vi "Read Event Details.vi"(1 "path":path, 2 "OK Button":bool, 3 "Event Name":string) -> (0 "text":string)   [LabVIEW 2014]
panel:
  out "error out":errorcluster
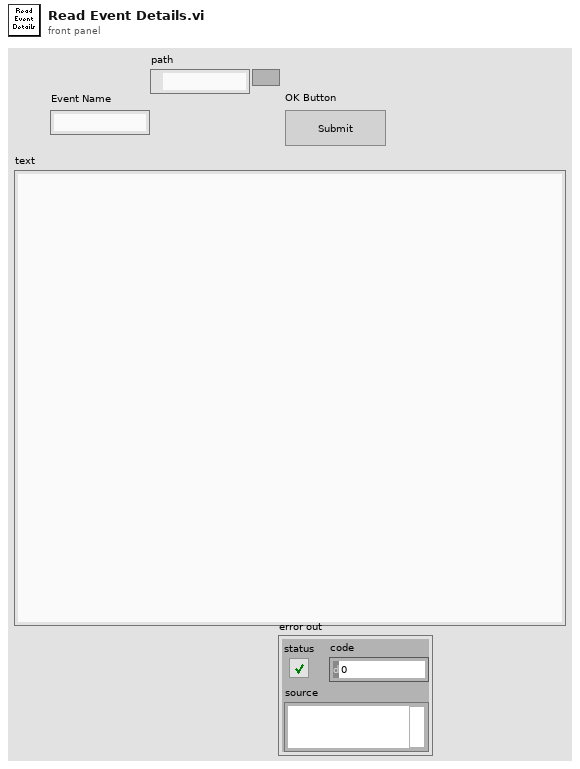
[diagram p1: front panel]
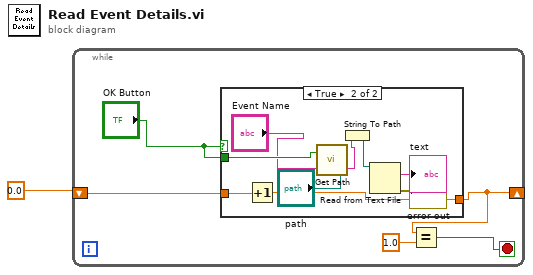
[diagram p0: block diagram]
diagram:
  n1 = while {
    shift-right: [w4] -> _
    shift-left: 0.0 ("Numeric") -> [w6]
    stop <- w5 stop-if-true
    n2 = case shown="True" "OK Button" {
      tunnel: w6 -> [w7 w14]
      tunnel: [w7 w13] -> w4
      tunnel: "OK Button" -> [_ w11]
      frame False {
      }
      frame True {
        n3 = Increment(x=w14) -> (x+1=w13:dbl)
        n4 = call "Get Path.vi"("path"="path", "Event Name"="Event Name", "OK Button"=w11) -> ("Event Location"=w9:string)
        n5 = String To Path(string=w9) -> (path=w16:path)
        n6 = Read from Text File(file (use dialog)=w16) -> (text=→"text":string, error out=→"error out":errorcluster)  [unwired: 3 in, 2 out]
      }
    }
    n7 = Equal?(x=w4, y=1.0) -> (x = y?=w5:bool)
  }
